vi "FGV_Timer.vi"(0 "Get Date/Time In Seconds":timestamp, 1 "Threshold Set":bool, 2 "Threshold":dbl, 5 "Start":bool, 7 "Pause":bool, 9 "Reset":bool, 11 "error in":errorcluster) -> (4 "Elapsed Time":dbl, 8 "Threshold Trigger":bool, 15 "error out":errorcluster)   [LabVIEW 2017]
doc: "This VI takes boolean Input of Time start, stop and reset. and additionally set threshold. \noutput of the VI is elapsed Time in seconds"
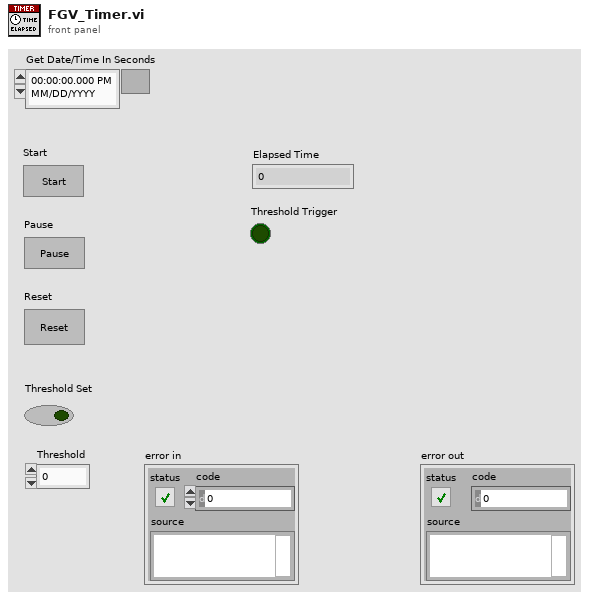
[diagram p1: front panel]
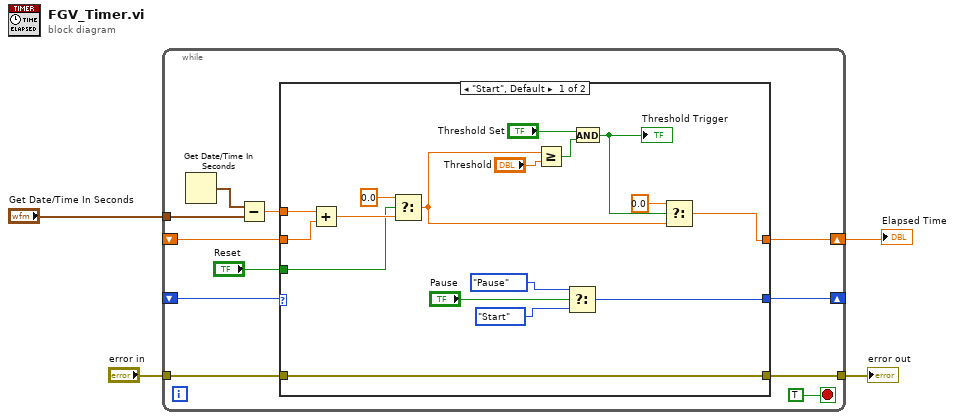
[diagram p0: block diagram]
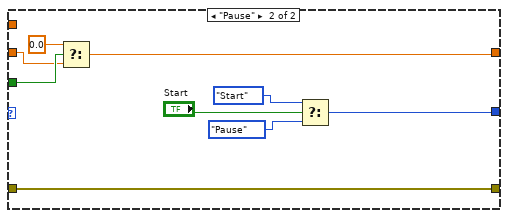
[diagram p2: hidden frame]
diagram:
  n1 = while {
    tunnel: "Get Date/Time In Seconds" -> [w12]
    shift-right: [w10] -> w3
    shift-left: _ -> [w9]
    shift-right: [w8] -> _
    shift-left: _ -> [w14]
    tunnel: "error in" -> [w6]
    tunnel: [w5] -> w1
    stop <- TRUE stop-if-true
    n2 = Get Date/Time In Seconds() -> (seconds since 1Jan1904=w13:timestamp)
    n3 = Subtract(x=w13, y=w12) -> (x-y=w11:dbl)
    n4 = case shown="\"Start\", Default" w14 {
      tunnel: w11 -> [w32 _]
      tunnel: [w17 w35] -> w10
      tunnel: w9 -> [w31 w34]
      tunnel: [w27 w38] -> w8
      tunnel: "Reset" -> [w24 w37]
      tunnel: w6 -> [w16 w33]
      tunnel: [w16 w33] -> w5
      frame "Start", Default {
        n5 = Add(x=w32, y=w31) -> (x+y=w26:dbl)
        n6 = Select(t=0.0, s=w24, f=w26) -> (s? t:f=w20:dbl)
        n7 = Greater Or Equal?(x=w20, y="Threshold") -> (x >= y?=w22:bool)
        n8 = Select(t=enum16{"Start", "Stop", "Pause", "Reset"}."Pause", s="Pause", f=enum16{"Start", "Stop", "Pause", "Reset"}."Start") -> (s? t:f=w27:enum16{"Start", "Stop", "Pause", "Reset"})
        n9 = And(x="Threshold Set", y=w22) -> (x .and. y?=w19:bool)
        "Threshold Trigger" <- w19
        n10 = Select(t=0.0, s=w19, f=w20) -> (s? t:f=w17:dbl)
      }
      frame "Pause" {
        n11 = Select(t=0.0, s=w37, f=w34) -> (s? t:f=w35:dbl)
        n12 = Select(t=enum16{"Start", "Stop", "Pause", "Reset"}."Start", s="Start", f=enum16{"Start", "Stop", "Pause", "Reset"}."Pause") -> (s? t:f=w38:enum16{"Start", "Stop", "Pause", "Reset"})
      }
    }
  }
  "Elapsed Time" <- w3
  "error out" <- w1
